vi "kuirs_机器视觉_卡尺测量_1.vi"() -> ()   [LabVIEW 2017]
uses:
  <vilib>/vision/NI_Vision_Development_Module.lvlib
panel:
  in  "旋转角度":dbl(slide) scale=0.0..180.0
  out "Edge Coordinates":cluster{"X":sgl, "Y":sgl}[](array[cluster]) {"Y" format="%.2f"; "X" format="%.2f"}
  out "Distance":sgl format="%.2f"
  out "原图":T1(plugin-control)
  in  "停止":bool
  out "模板":T1(plugin-control)
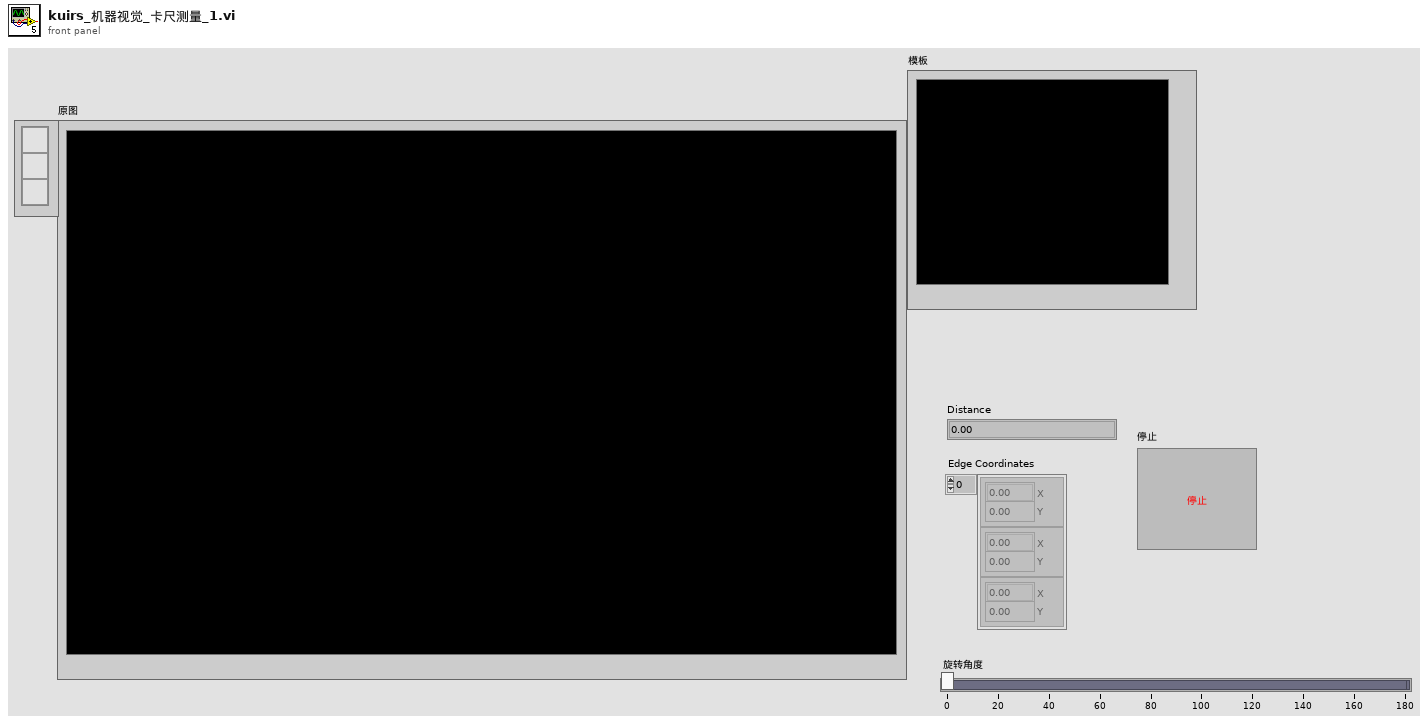
[diagram p1: front panel]
types:
  T1 = typedef "IMAQ Image.ctl" = refnum<image>
  T2 = typedef "Image Type" = u32
  T3 = typedef "IMAQ Rectangle" = cluster{"Left":i32, "Top":i32, "Right":i32, "Bottom":i32, "Rotation":dbl}
  T4 = typedef "ROI Descriptor" = cluster{"Global Rectangle":i32[], "Contours":cluster{"ID":enum32{"External", "Internal"}, "Type":u32, "Coordinates":i32[]}[]}
  T5 = cluster{"Global Rectangle":i32[], "Contours":cluster{"Contour Type":u32, "ROI Type":u32, "Points":i32[]}[]}
  T6 = cluster{"Contrast":i32, "Filter width":i32, "Steepness":i32, "Subsampling Ratio":u32, "Show Search Area":bool, "Show Search Lines":bool, "Show Edges Found":bool, "Show Result":bool}
  T7 = typedef "IMAQ Coordinate System" = cluster{"Reference System":cluster{"Origin":cluster{"X":sgl, "Y":sgl}, "Angle (deg)":sgl, "Axis Reference":u32}, "Measurement System":cluster{"Origin":cluster{"X":sgl, "Y":sgl}, "Angle (deg)":sgl, "Axis Reference":u32}}
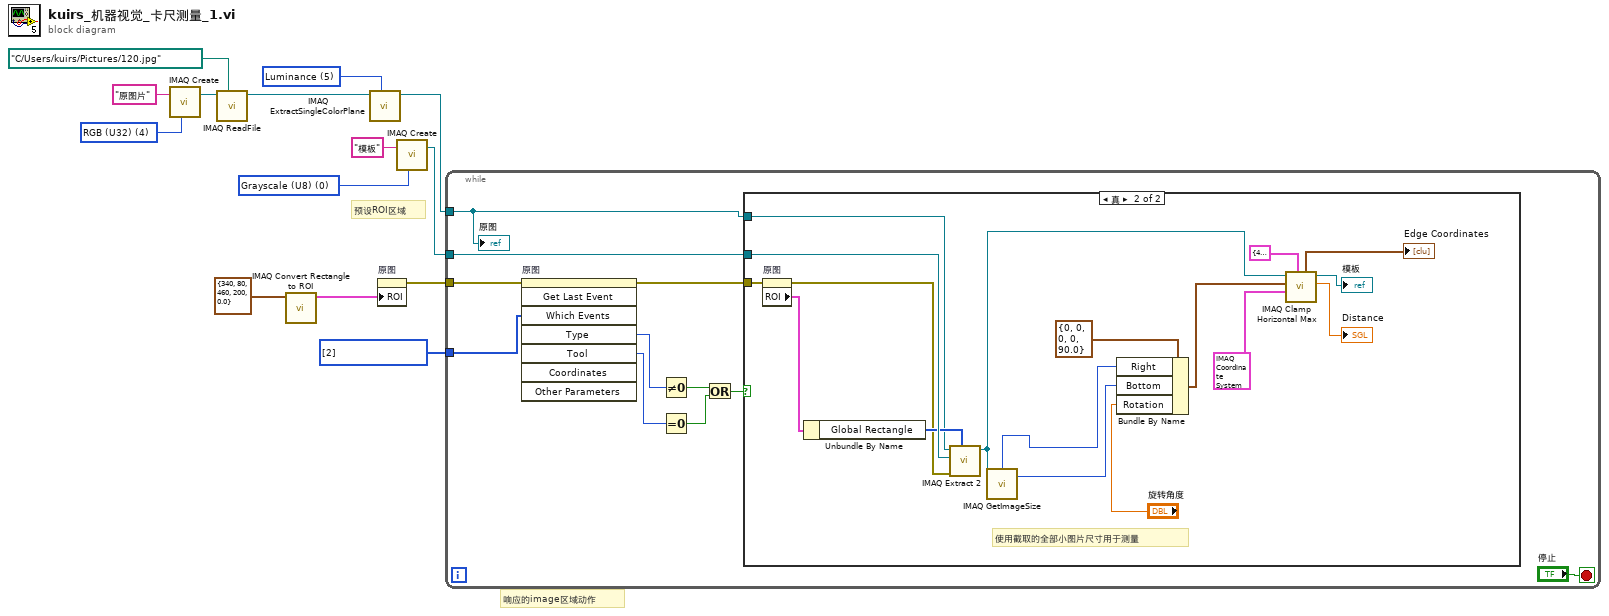
[diagram p0: block diagram]
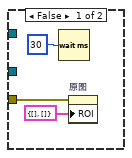
[diagram p2: hidden frame]
diagram:
  w3 = T2 0 items=["Grayscale (U8)", "Grayscale (I16)", "Grayscale (SGL)", "Complex (CSG)", "RGB (U32)", "HSL (U32)", "RGB (U64)", "Grayscale (U16)"] ("Image Type")
  w4 = i32[] [2] items=["No Event"=0, "Click Event"=1, "Draw Event"=2, "Size Event"=4, "Scroll Event"=5, "Double Click Event"=8] ("Which Events")
  w9 = 5 items=["Red", "Green", "Blue", "Hue", "Saturation", "Luminance", "Value", "Intensity"] ("Color Plane")
  w11 = T2 4 items=["Grayscale (U8)", "Grayscale (I16)", "Grayscale (SGL)", "Complex (CSG)", "RGB (U32)", "HSL (U32)", "RGB (U64)", "Grayscale (U16)"] ("Image Type")
  # "响应的image区域动作"
  # "预设ROI区域"
  n1 = call "IMAQ Create"("Image Name"="原图片", "Image Type"=w11) -> ("New Image"=w13:T1)  [unwired: 3 in, 1 out]
  n2 = call "IMAQ ReadFile"("File Path"=path "C:/Users/kuirs/Pictures/120.jpg", "Image"=w13) -> ("Image Out"=w10:T1)  [unwired: 5 in, 4 out]
  n3 = call "IMAQ Convert Rectangle to ROI"("Rectangle"=T3 {"Left"=340, "Top"=80, "Right"=460, "Bottom"=200, "Rotation"=0.0}) -> ("ROI Descriptor"=w6:T4)  [unwired: 8 in, 1 out]
  n4 = call "IMAQ ExtractSingleColorPlane"("Color Plane"=w9, "Image Src"=w10) -> ("Image Dst Out"=w8:T1)  [unwired: 8 in, 1 out]
  n5 = property on="原图" class="ImageControl"("ROI"=w6) -> (error out=w5:errorcluster)  [unwired: 2 in, 1 out]
  n6 = call "IMAQ Create"("Image Name"="模板", "Image Type"=w3) -> ("New Image"=w1:T1)  [unwired: 3 in, 1 out]
  n7 = while {
    tunnel: w8 -> [w15]
    tunnel: w5 -> [w24]
    tunnel: w4 -> [w23]
    tunnel: w1 -> [w16]
    stop <- "停止" stop-if-true
    n8 = invoke on="原图" class="ImageControl" method="Get Last Event"(error in=w24, "Which Events"=w23) -> (error out=w22:errorcluster, "Type"=w21:i32, "Tool"=w20:i32)  [unwired: 6 in, 5 out]
    n9 = Not Equal To 0?(x=w21) -> (x != 0?=w19:bool)
    n10 = Equal To 0?(x=w20) -> (x = 0?=w18:bool)
    n11 = Or(x=w19, y=w18) -> (x .or. y?=w17:bool)
    n12 = case shown="真" w17 {
      tunnel: w22 -> [w27 w45]
      tunnel: w16 -> [_ w43]
      tunnel: w15 -> [_ w41]
      frame False {
        n13 = Wait (ms)(milliseconds to wait=u32 30 ("等待时间（毫秒）")) -> ()  [unwired: 1 out]
        n14 = property on="原图" class="ImageControl"(error in=w27, "ROI"=T5 {"Global Rectangle"=[], "Contours"=[]}) -> ()  [unwired: 1 in, 2 out]
      }
      frame True {
        # "使用截取的全部小图片尺寸用于测量"
        n15 = property on="原图" class="ImageControl"(error in=w45) -> (error out=w40:errorcluster, "ROI"=w44:T5)  [unwired: 1 in, 1 out]
        n16 = Unbundle By Name(w44) -> ("Global Rectangle"=w42:i32[])
        n17 = call "IMAQ Extract 2"("Optional Rectangle"=w42, "error in (no error)"=w40, "Image Dst"=w43, "Image Src"=w41) -> ("Image Dst Out"=w37:T1)  [unwired: 6 in, 1 out]
        n18 = call "IMAQ GetImageSize"("Image"=w37) -> ("Y Resolution"=w34:i32, "X Resolution"=w35:i32)  [unwired: 3 in, 1 out]
        n19 = Bundle By Name(cluster=T3 {"Left"=0, "Top"=0, "Right"=0, "Bottom"=0, "Rotation"=90.0} ("Rectangle"), "Right"=w35, "Bottom"=w34, "Rotation"="旋转角度") -> (w33:T3)
        n20 = call "IMAQ Clamp Horizontal Max"("Settings"=T6 {"Contrast"=40, "Filter width"=4, "Steepness"=2, "Subsampling Ratio"=5, "Show Search Area"=TRUE, "Show Search Lines"=TRUE, "Show Edges Found"=TRUE, "Show Result"=TRUE}, "Coordinate System"=T7 {"Reference System"={"Origin"={"X"=0.0, "Y"=0.0}, "Angle (deg)"=0.0, "Axis Reference"=0}, "Measurement System"={"Origin"={"X"=0.0, "Y"=0.0}, "Angle (deg)"=0.0, "Axis Reference"=0}}, "Rectangle"=w33, "Image"=w37) -> ("Distance"=→"Distance":sgl, "Image Out"=→"模板":T1, "Edge Coordinates"=→"Edge Coordinates":cluster{"X":sgl, "Y":sgl}[])  [unwired: 3 in, 2 out]
      }
    }
    "原图" <- w15
  }
